vi "Create Front Panel Events.vi"(8 "error in (no error)":errorcluster, 11 "Main Window in":refnum<class "Main Window.lvclass">) -> (0 "error out":errorcluster, 3 "Main Window out":refnum<class "Main Window.lvclass">)   [LabVIEW 2023, in "Main Window.lvlib" / "Main Window.lvclass"]
uses:
  Main Window.lvclass
  Main Window.lvclass/Main Window.ctl
  Application/Mode.ctl
  Application/Application.lvlib
  UI Window/UI Window.lvclass
  Hardware/Autosampler/Autosampler State.ctl
  Hardware/Autosampler/Autosampler.lvlib
  Hardware/Autosampler/Autosampler Status.ctl
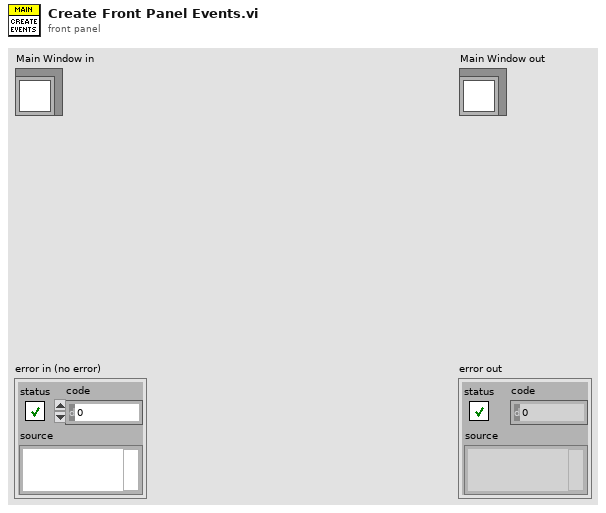
[diagram p1: front panel]
types:
  T1 = typedef "Autosampler.lvlib/Autosampler Status.ctl" = cluster{"State":T2, "Valve Position":u16, "Well index":u16, "Fill Volume":u16, "Needle Position":enum16{"Home", "Well", "Wash Port"}}
  T2 = typedef "Autosampler.lvlib/Autosampler State.ctl" = enum16{"Ready", "Injection", "Washing", "Shaking", "Getting Ready", "Error"}
  T3 = typedef "Application.lvlib/Mode.ctl" = enum16{"Idle", "Cancel", "Live", "Stream", "Autofocus", "Z-Stack", "Montage", "Saving", "Stage Scan", "Laser Adjust"}
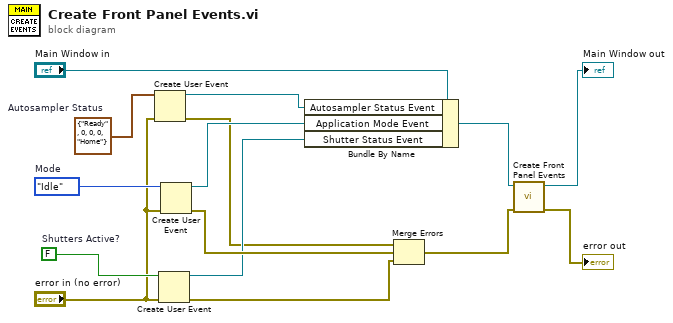
[diagram p0: block diagram]
diagram:
  w2 = T1 {"State"=enum."Ready", "Valve Position"=0, "Well index"=0, "Fill Volume"=0, "Needle Position"=enum."Home"}  # Autosampler Status
  w6 = FALSE  # Shutters Active?
  w11 = Mode."Idle"  # Mode
  n1 = Create User Event(user event datatype=w2, error in="error in (no error)") -> (user event=w1:refnum<user-event>, error out=w3:errorcluster)
  n2 = Create User Event(user event datatype=w6, error in="error in (no error)") -> (user event=w5:refnum<user-event>, error out=w7:errorcluster)
  n3 = Create User Event(user event datatype=w11, error in="error in (no error)") -> (user event=w10:refnum<user-event>, error out=w8:errorcluster)
  n4 = Bundle By Name(cluster="Main Window in", "Autosampler Status Event"=w1, "Application Mode Event"=w10, "Shutter Status Event"=w5) -> (w12:refnum<class "Main Window.lvclass">)
  n5 = Merge Errors(w3, w8, w7) -> (w9:errorcluster)
  n6 = call-parent "Create Front Panel Events.vi"("error in (no error)"=w9, "UI Window in"=w12) -> ("error out"=→"error out":errorcluster, "UI Window out"=→"Main Window out":refnum<class "Main Window.lvclass">)  [unwired: 8 in]
